vi "FTW-Example-SQLite.vi"() -> ()   [LabVIEW 2012]
uses:
  Core/src/Database/FTW-SQLite-DatabaseType.ctl
  Core/src/Time/FTW-Time-Uptime.vi
  Core/src/Database/FTW-SQLite-PrepareStatement.vi
  Core/src/Database/FTW-SQLite-LibraryFilepath.vi
  Core/src/Database/FTW-SQLite-LibraryReturnValue.vi
  Core/src/Error/FTW-ERR-ThrowImpossibleError.vi
  Core/utils/CodeGen/SQLite-Fetch/FTW-SQLite-Fetch.xnode
  Core/src/Database/FTW-SQLite-Connector.lvclass
  Core/src/Database/FTW-SQLite-AccessMode.ctl
panel:
  out "Result Set":cluster{"Year":string}[](array[cluster])
  out "Time to Compile SQL (Fetch)":dbl format="%.6fsec"
  out "Time to Execute+Compile (Fetch)":dbl format="%.6fsec"
  out "Time to Compile SQL (DDL)":dbl format="%.6fsec"
  out "Time to Execute+Compile (DDL)":dbl format="%.6fsec"
  out "Results from Database":T1(array[cluster])
  out "Data to put into Database":T2(array[cluster])
  out "error out":errorcluster
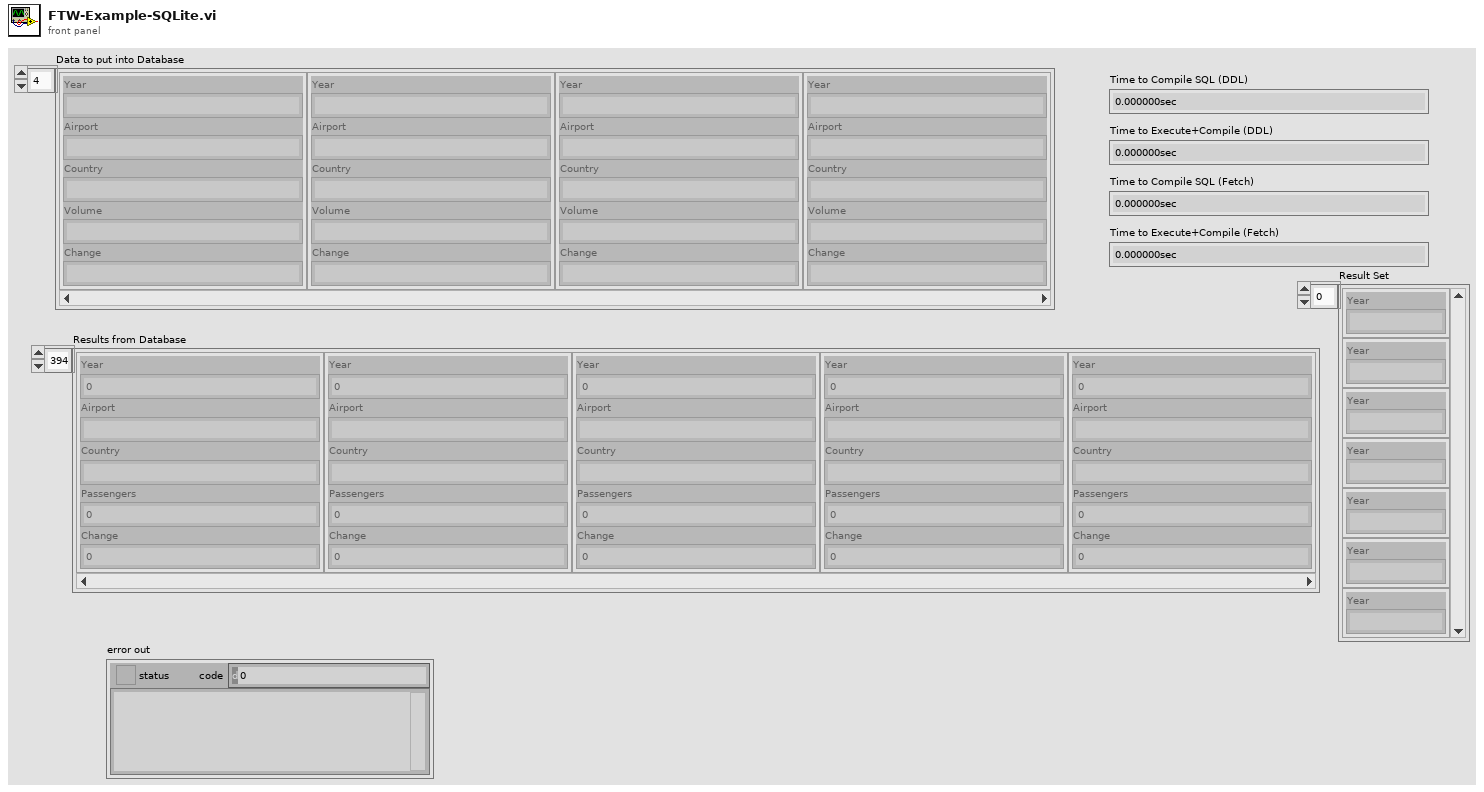
[diagram p1: front panel]
types:
  T1 = cluster{"Year":i32, "Airport":string, "Country":string, "Passengers":i32, "Change":dbl}[]
  T2 = cluster{"Year":string, "Airport":string, "Country":string, "Volume":string, "Change":string}[]
  T3 = cluster{"Year":i32, "Airport":string, "Country":string, "Passengers":i32, "Change":dbl}
  T4 = cluster{"Year":string, "Airport":string, "Country":string, "Volume":string, "Change":string}
  T5 = typedef "FTW-SQLite-Connector.lvclass/FTW-SQLite-DatabaseType.ctl" = enum16{"Disk", "Memory"}
  T6 = typedef "FTW-SQLite-Connector.lvclass/FTW-SQLite-AccessMode.ctl" = enum16{"Read", "Read/Write", "Read/Write/Create"}
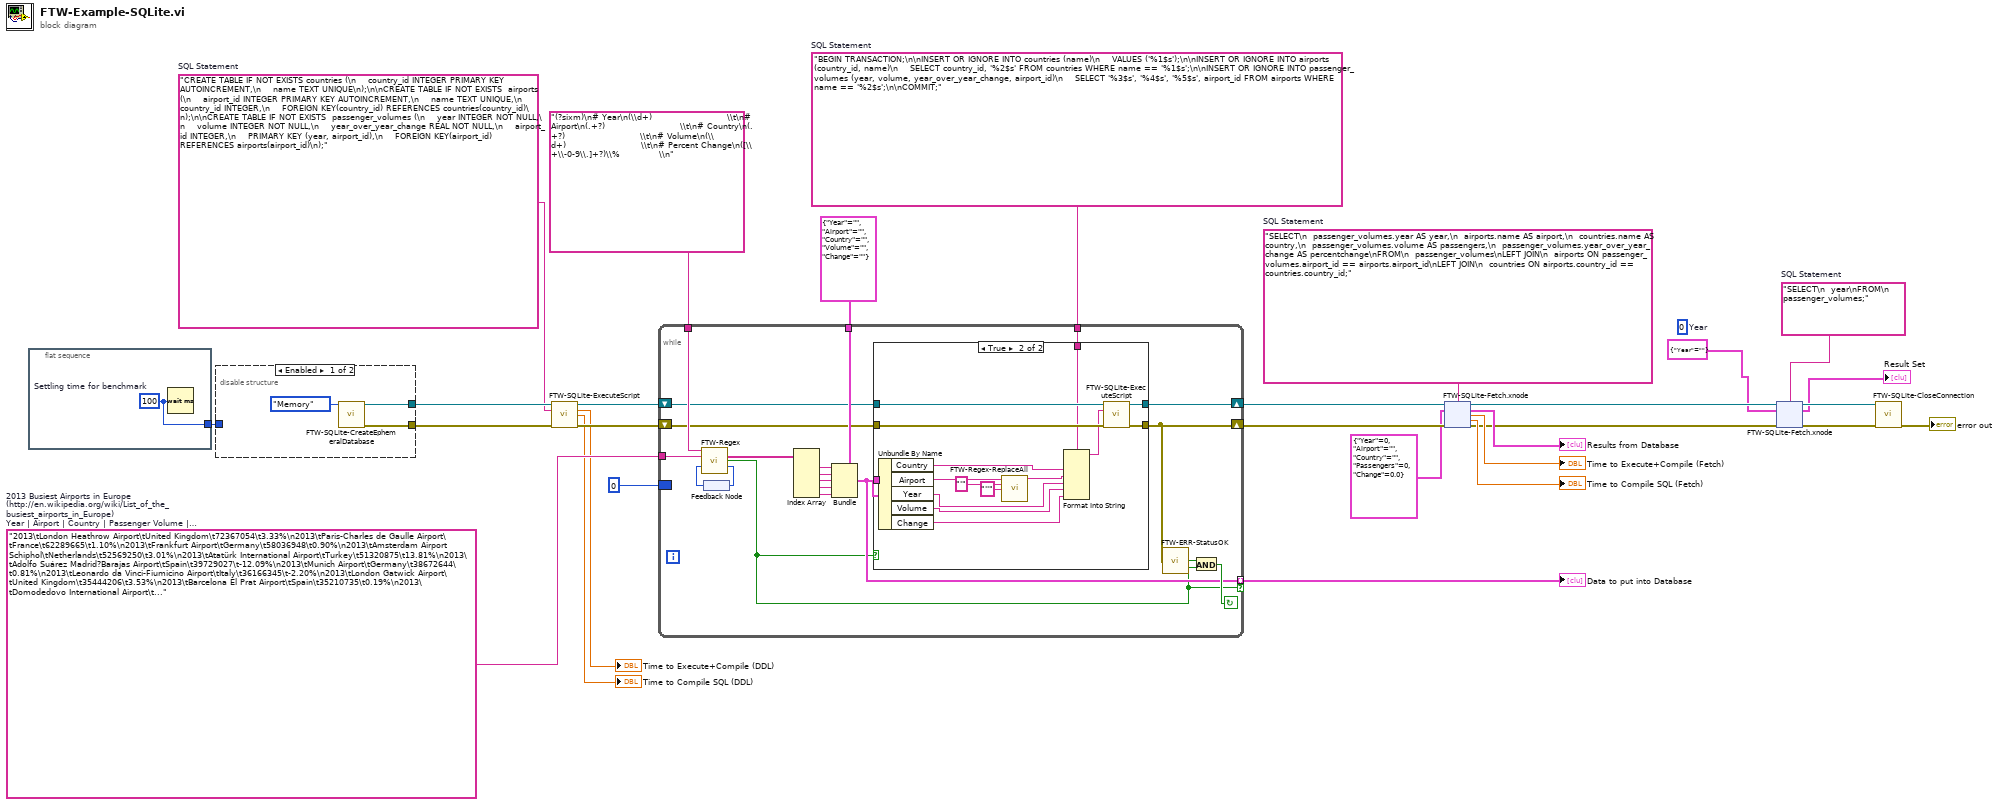
[diagram p0: block diagram]
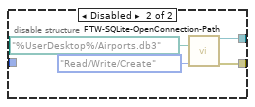
[diagram p2: hidden frame]
diagram:
  (unwired) 0  # Year
  w4 = "SELECT\n  year\nFROM\n  passenger_volumes;"  # SQL Statement
  w16 = "SELECT\n  passenger_volumes.year AS year,\n  airports.name AS airport,\n  countries.name AS country,\n  passenger_volumes.volume AS passengers,\n  passenger_volumes.year_over_year_change AS percentchange\nFROM\n  passenger_volumes\nLEFT JOIN\n  airports ON passenger_volumes.airport_id == airports.airport_id\nLEFT JOIN\n  countries ON airports.country_id == countries.country_id;"  # SQL Statement
  w19 = "BEGIN TRANSACTION;\n\nINSERT OR IGNORE INTO countries (name)\n    VALUES ('%1$s');\n\nINSERT OR IGNORE INTO airports (country_id, name)\n    SELECT country_id, '%2$s' FROM countries WHERE name == '%1$s';\n\nINSERT OR IGNORE INTO passenger_volumes (year, volume, year_over_year_change, airport_id)\n    SELECT '%3$s', '%4$s', '%5$s', airport_id FROM airports WHERE name == '%2$s';\n\nCOMMIT;"  # SQL Statement
  w25 = "2013\tLondon Heathrow Airport\tUnited Kingdom\t72367054\t3.33%\n2013\tParis-Charles de Gaulle Airport\tFrance\t62289665\t1.10%\n2013\tFrankfurt Airport\tGermany\t58036948\t0.90%\n2013\tAmsterdam Airport Schiphol\tNetherlands\t52569250\t3.01%\n2013\tAtatürk International Airport\tTurkey\t51320875\t13.81%\n2013\tAdolfo Suárez Madrid?Barajas Airport\tSpain\t39729027\t-12.09%\n2013\tMunich Airport\tGermany\t38672644\t0.81%\n2013\tLeonardo da Vinci-Fiumicino Airport\tItaly\t36166345\t-2.20%\n2013\tLondon Gatwick Airport\tUnited Kingdom\t35444206\t3.53%\n2013\tBarcelona El Prat Airport\tSpain\t35210735\t0.19%\n2013\tDomodedovo International Airport\tRussia\t30760000\t9.21%\n2013\tSheremetyevo International Airport\tRussia\t29256000\t12.38%\n2013\tParis-Orly Airport\tFrance\t28274154\t3.83%\n2013\tAntalya Airport\tTurkey\t27003712\t8.04%\n2013\tZürich Airport\tSwitzerland\t24865138\t0.25%\n2013\tCopenhagen Airport, Kastrup\tDenmark\t24067030\t3.13%\n2013\tOslo Gardermoen International Airport\tNorway\t22956540\t3.97%\n2013\tPalma de Mallorca Airport\tSpain\t22768082\t0.45%\n2013\tVienna International Airport\tAustria\t21999926\t-0.75%\n2013\tDüsseldorf International Airport\tGermany\t21228226\t1.90%\n2013\tManchester Airport\tUnited Kingdom\t20751581\t5.14%\n2013\tStockholm-Arlanda Airport\tSweden\t20681554\t5.29%\n2013\tDublin Airport\tIreland\t20200000\t5.76%\n2013\tBerlin Tegel Airport\tGermany\t19591838\t7.86%\n2013\tBrussels Airport\tBelgium\t19133222\t0.85%\n2013\tSabiha Gökçen Airport\tTurkey\t18641842\t28.68%\n2013\tMalpensa Airport\tItaly\t17955075\t-3.14%\n2013\tLondon Stansted Airport\tUnited Kingdom\t17852393\t2.17%\n2013\tLisbon Portela Airport\tPortugal\t16024955\t4.73%\n2013\tHelsinki-Vantaa Airport\tFinland\t15279043\t2.83%\n2013\tGeneva International Airport\tSwitzerland\t14436149\t3.86%\n2013\tHamburg Airport\tGermany\t13502553\t-1.42%\n2013\tMálaga Airport\tSpain\t12922403\t2.71%\n2013\tPulkovo Airport\tRussia\t12854366\t15.24%\n2013\tAthens International Airport\tGreece\t12460298\t-3.74%\n2013\tNice Côte d'Azur Airport\tFrance\t11554195\t3.26%\n2013\tVnukovo International Airport\tRussia\t11180000\t15.38%\n2013\tVáclav Havel Airport Prague\tCzech Republic\t10974196\t1.54%\n2013\tEsenbo?a International Airport\tTurkey\t10928403\t18.30%\n2013\tFrederic Chopin Airport\tPoland\t10683402\t11.43%\n2013\tAdnan Menderes Airport\tTurkey\t10208627\t9.11%\n2013\tEdinburgh Airport\tUnited Kingdom\t9775443\t6.31%\n2013\tGran Canaria Airport\tSpain\t9770253\t-1.23%\n2013\tLondon Luton Airport\tUnited Kingdom\t9697944\t0.83%\n2013\tAlicante Airport\tSpain\t9638860\t8.85%\n2013\tStuttgart Airport\tGermany\t9577551\t-1.47%\n2013\tBirmingham Airport\tUnited Kingdom\t9120201\t2.22%\n2013\tCologne Bonn Airport\tGermany\t9077346\t-2.18%\n2013\tLinate Airport\tItaly\t9034373\t-2.12%\n2013\tOrio al Serio Airport\tItaly\t8964376\t0.83%\n2013\tTenerife South Airport\tSpain\t8701983\t2.01%\n2013\tLyon-Saint Exupéry Airport\tFrance\t8562288\t1.32%\n2013\tBudapest Liszt Ferenc International Airport\tHungary\t8520880\t0.20%\n2013\tVenice Marco Polo Airport\tItaly\t8403790\t2.63%\n2013\tMarseille Provence Airport\tFrance\t8260619\t-0.42%\n2013\tBoryspil International Airport\tUkraine\t7930000\t-6.46%\n2013\tHenri Coand? International Airport\tRomania\t7649503\t7.44%\n2013\tBlagnac Airport\tFrance\t7567634\t0.11%\n2013\tGlasgow International Airport\tUnited Kingdom\t7363764\t2.88%\n2013\tBrussels South Charleroi Airport\tBelgium\t6786979\t4.15%\n2013\tBerlin Schönefeld Airport\tGermany\t6727306\t-5.21%\n2013\tCatania-Fontanarossa Airport\tItaly\t6400127\t2.45%\n2013\tFrancisco de Sá Carneiro Airport\tPortugal\t6370749\t5.30%\n2013\tBergen Flesland Airport\tNorway\t6213960\t6.87%\n2013\tBologna Airport\tItaly\t6193783\t3.95%\n2013\tBristol Airport\tUnited Kingdom\t6131896\t3.55%\n2013\tFaro Airport\tPortugal\t5978685\t5.40%\n2013\tEuroAirport Basel-Mulhouse-Freiburg\tSwitzerland-France-Germany\t5880771\t9.83%\n2013\tHeraklion International Airport\tGreece\t5792429\t15.52%\n2013\tIbiza Airport\tSpain\t5726581\t3.09%\n2013\tNaples Airport\tItaly\t5444422\t-6.16%\n2013\tLanzarote Airport\tSpain\t5334598\t3.21%\n2013\tLangenhagen Airport\tGermany\t5234909\t-1.00%\n2013\tGothenburg-Landvetter Airport\tSweden\t5004093\t3.07%\n2013\tLarnaca International Airport\tCyprus\t4863577\t-5.86%\n2013\tRiga International Airport\tLatvia\t4793213\t0.53%\n2013\tRome Ciampino Airport\tItaly\t4749251\t5.60%\n2013\tStavanger Sola Airport\tNorway\t4668403\t5.76%\n2013\tValencia Airport\tSpain\t4599990\t-3.20%\n2013\tBordeaux - Mérignac Airport\tFrance\t4574357\t4.43%\n2013\tGalileo Galilei Airport\tItaly\t4479690\t-0.34%\n2013\tNewcastle Airport\tUnited Kingdom\t4420839\t1.25%\n2013\tPalermo Airport\tItaly\t4349672\t-5.62%\n2013\tEast Midlands Airport\tUnited Kingdom\t4334117\t6.33%\n2013\tAdana ?akirpa?a Airport\tTurkey\t4316678\t14.28%\n2013\tTrondheim Værnes Airport\tNorway\t4311328\t3.63%\n2013\tKoltsovo Airport\tRussia\t4293002\t13.48%\n2013\tFuerteventura Airport\tSpain\t4259341\t-3.18%\n2013\tRhodes International Airport\tGreece\t4200068\t10.10%\n2013\tLiverpool John Lennon Airport\tUnited Kingdom\t4187493\t-6.18%\n2013\tThessaloniki International Airport, \"Macedonia\"\tGreece\t4085032\t1.05%\n2013\tDalaman Airport\tTurkey\t4057173\t6.49%\n2013\tMalta International Airport\tMalta\t4052000\t10.88%\n2013\tBelfast International Airport\tUnited Kingdom\t4023336\t-6.73%\n2013\tBeauvais-Tillé Airport\tFrance\t3952908\t2.34%\n2013\tNantes Atlantique Airport\tFrance\t3930849\t8.24%\n2013\tBilbao Airport\tSpain\t3800789\t-8.88%\n2013\tTolmachevo Airport\tRussia\t3748211\t14.74%\n2013\tSan Pablo Airport\tSpain\t3687727\t-14.08%\n2013\tKraków Airport\tPoland\t3647616\t6.07%\n2012\tLondon Heathrow Airport\tUnited Kingdom\t70037417\t0.87%\n2012\tParis-Charles de Gaulle Airport\tFrance\t61611934\t1.05%\n2012\tFrankfurt Airport\tGermany\t57520001\t1.92%\n2012\tAmsterdam Airport Schiphol\tNetherlands\t51035590\t2.57%\n2012\tMadrid?Barajas Airport\tSpain\t45190528\t-9.02%\n2012\tAtatürk International Airport\tTurkey\t45091962\t20.58%\n2012\tMunich Airport\tGermany\t38360604\t1.58%\n2012\tLeonardo da Vinci-Fiumicino Airport\tItaly\t36980911\t-1.78%\n2012\tBarcelona El Prat Airport\tSpain\t35144503\t2.17%\n2012\tLondon Gatwick Airport\tUnited Kingdom\t34235982\t1.67%\n2012\tDomodedovo International Airport\tRussia\t28165657\t9.59%\n2012\tParis-Orly Airport\tFrance\t27232263\t0.34%\n2012\tSheremetyevo International Airport\tRussia\t26032975\t16.47%\n2012\tAntalya Airport\tTurkey\t24993667\t-0.48%\n2012\tZürich Airport\tSwitzerland\t24802466\t1.91%\n2012\tCopenhagen Airport, Kastrup\tDenmark\t23336187\t2.69%\n2012\tPalma de Mallorca Airport\tSpain\t22666858\t-0.26%\n2012\tVienna International Airport\tAustria\t22165794\t5.02%\n2012\tOslo Gardermoen International Airport\tNorway\t22080433\t4.63%\n2012\tDüsseldorf International Airport\tGermany\t20833246\t2.43%\n2012\tManchester Airport\tUnited Kingdom\t19736502\t4.47%\n2012\tStockholm-Arlanda Airport\tSweden\t19642029\t3.00%\n2012\tDublin Airport\tIreland\t19099649\t1.91%\n2012\tBrussels Airport\tBelgium\t18971332\t0.99%\n2012\tMalpensa Airport\tItaly\t18537301\t-3.97%\n2012\tBerlin Tegel Airport\tGermany\t18164203\t7.35%\n2012\tLondon Stansted Airport\tUnited Kingdom\t17472699\t-3.21%\n2012\tLisbon Portela Airport\tPortugal\t15301176\t3.35%\n2012\tHelsinki Airport\tFinland\t14858215\t-0.05%\n2012\tSabiha Gökçen Airport\tTurkey\t14487242\t13.63%\n2012\tGeneva International Airport\tSwitzerland\t13899422\t6.01%\n2012\tHamburg Airport\tGermany\t13697402\t1.03%\n2012\tAthens International Airport\tGreece\t12944041\t-10.40%\n2012\tMálaga Airport\tSpain\t12581944\t-1.88%\n2012\tNice Côte d'Azur Airport\tFrance\t11189896\t7.37%\n2012\tPulkovo Airport\tRussia\t11154560\t16.06%\n2012\tVáclav Havel Airport Prague\tCzech Republic\t10807890\t-8.32%\n2012\tGran Canaria Airport\tSpain\t9892067\t-6.14%\n2012\tStuttgart Airport\tGermany\t9720877\t1.45%\n2012\tVnukovo International Airport\tRussia\t9690000\t18.21%\n2012\tLondon Luton Airport\tUnited Kingdom\t9617697\t1.09%\n2012\tFrederic Chopin Airport\tPoland\t9587842\t2.68%\n2012\tAdnan Menderes Airport\tTurkey\t9356284\t9.77%\n2012\tCologne Bonn Airport\tGermany\t9280070\t-3.57%\n2012\tEsenbo?a Airport\tTurkey\t9237886\t8.87%\n2012\tLinate Airport\tItaly\t9229890\t1.11%\n2012\tEdinburgh Airport\tUnited Kingdom\t9195061\t-2.03%\n2012\tBirmingham Airport\tUnited Kingdom\t8922539\t3.55%\n2012\tOrio al Serio Airport\tItaly\t8890720\t5.59%\n2012\tAlicante Airport\tSpain\t8855444\t-10.67%\n2012\tTenerife South Airport\tSpain\t8530729\t-1.45%\n2012\tBudapest Liszt Ferenc International Airport\tHungary\t8504020\t-4.67%\n2012\tBoryspil International Airport\tUkraine\t8478091\t5.36%\n2012\tLyon-Saint Exupéry Airport\tFrance\t8451039\t0.16%\n2012\tMarseille Provence Airport\tFrance\t8295479\t12.61%\n2012\tVenice Marco Polo Airport\tItaly\t8188455\t-4.62%\n2012\tBlagnac Airport\tFrance\t7559350\t8.17%\n2012\tGlasgow International Airport\tUnited Kingdom\t7157859\t4.04%\n2012\tHenri Coand? International Airport\tRomania\t7120067\t41.01%\n2012\tBerlin Schönefeld Airport\tGermany\t7097274\t-0.23%\n2012\tBrussels South Charleroi Airport\tBelgium\t6516427\t10.43%\n2012\tCatania-Fontanarossa Airport\tItaly\t6246888\t-8.05%\n2012\tFrancisco de Sá Carneiro Airport\tPortugal\t6050094\t0.76%\n2012\tBologna Airport\tItaly\t5958648\t1.24%\n2012\tBristol Airport\tUnited Kingdom\t5921530\t2.44%\n2012\tBergen Flesland Airport\tNorway\t5814413\t3.80%\n2012\tNaples Airport\tItaly\t5801836\t0.57%\n2012\tFaro Airport\tPortugal\t5672377\t1.01%\n2012\tIbiza Airport\tSpain\t5555048\t-1.56%\n2012\tEuroAirport Basel-Mulhouse-Freiburg\tSwitzerland-France-Germany\t5354674\t5.96%\n2012\tLangenhagen Airport\tGermany\t5287831\t-0.98%\n2012\tLanzarote Airport\tSpain\t5168775\t-6.76%\n2012\tLarnaca International Airport\tCyprus\t5166224\t-6.20%\n2012\tHeraklion International Airport\tGreece\t5014312\t-5.26%\n2012\tGothenburg-Landvetter Airport\tSweden\t4854888\t-1.05%\n2012\tRiga International Airport\tLatvia\t4767878\t-6.64%\n2012\tValencia Airport\tSpain\t4752020\t-4.57%\n2012\tPalermo Airport\tItaly\t4608533\t-7.70%\n2012\tRome Ciampino Airport\tItaly\t4497376\t-5.95%\n2012\tGalileo Galilei Airport\tItaly\t4494915\t-0.70%\n2012\tLiverpool John Lennon Airport\tUnited Kingdom\t4463257\t-15.00%\n2012\tStavanger Sola Airport\tNorway\t4413987\t6.83%\n2012\tFuerteventura Airport\tSpain\t4399023\t-11.10%\n2012\tBordeaux - Mérignac Airport\tFrance\t4380145\t6.38%\n2012\tNewcastle Airport\tUnited Kingdom\t4366196\t0.46%\n2012\tBelfast International Airport\tUnited Kingdom\t4313685\t5.12%\n2012\tSan Pablo Airport\tSpain\t4292020\t-13.46%\n2012\tBilbao Airport\tSpain\t4171065\t3.09%\n2012\tTrondheim Værnes Airport\tNorway\t4160162\t5.95%\n2012\tEast Midlands Airport\tUnited Kingdom\t4076178\t-3.30%\n2012\tThessaloniki International Airport, \"Macedonia\"\tGreece\t4042539\t-0.47%\n2012\tBeauvais-Tillé Airport\tFrance\t3862431\t5.02%\n2012\tRhodes International Airport\tGreece\t3814706\t-8.06%\n2012\tDalaman Airport\tTurkey\t3810015\t2.06%\n2012\tKoltsovo Airport\tRussia\t3783069\t12.73%\n2012\tBari Airport\tItaly\t3780112\t1.46%\n2012\tAdana ?akirpa?a Airport\tTurkey\t3777348\t16.55%\n2012\tLos Rodeos Airport\tSpain\t3717944\t-9.21%\n2012\tMalta International Airport\tMalta\t3654283\t4.10%\n2012\tNantes Atlantique Airport\tFrance\t3631693\t11.88%\n2011\tLondon Heathrow Airport\tUnited Kingdom\t69433230\t5.39%\n2011\tParis-Charles de Gaulle Airport\tFrance\t60970551\t4.82%\n2011\tFrankfurt Airport\tGermany\t56436255\t6.46%\n2011\tAmsterdam Airport Schiphol\tNetherlands\t49755252\t10.05%\n2011\tMadrid Barajas Airport\tSpain\t49671270\t-0.39%\n2011\tMunich Airport\tGermany\t37763701\t8.76%\n2011\tRome-Fiumicino Airport\tItaly\t37651700\t3.62%\n2011\tAtatürk International Airport\tTurkey\t37394694\t16.34%\n2011\tBarcelona El Prat Airport\tSpain\t34398226\t17.76%\n2011\tLondon Gatwick Airport\tUnited Kingdom\t33674264\t7.33%\n2011\tParis-Orly Airport\tFrance\t27139076\t7.68%\n2011\tDomodedovo International Airport\tRussia\t25701610\t15.49%\n2011\tAntalya Airport\tTurkey\t25113635\t14.09%\n2011\tZurich Airport\tSwitzerland\t24337954\t6.38%\n2011\tPalma de Mallorca Airport\tSpain\t22726707\t7.62%\n2011\tCopenhagen Airport\tDenmark\t22725517\t5.69%\n2011\tSheremetyevo International Airport\tRussia\t22351317\t16.88%\n2011\tVienna International Airport\tAustria\t21106292\t7.19%\n2011\tOslo-Gardermoen Airport\tNorway\t21103623\t10.54%\n2011\tDüsseldorf International Airport\tGermany\t20339466\t7.12%\n2011\tMilan Malpensa Airport\tItaly\t19303131\t1.88%\n2011\tStockholm-Arlanda Airport\tSweden\t19069065\t12.42%\n2011\tManchester Airport\tUnited Kingdom\t18892756\t6.38%\n2011\tBrussels Airport\tBelgium\t18786034\t9.34%\n2011\tDublin Airport\tIreland\t18740593\t1.68%\n2011\tLondon Stansted Airport\tUnited Kingdom\t18052843\t-2.80%\n2011\tBerlin Tegel Airport\tGermany\t16919820\t12.61%\n2011\tHelsinki Airport\tFinland\t14865871\t15.39%\n2011\tLisbon Portela Airport\tPortugal\t14805624\t5.49%\n2011\tAthens International Airport\tGreece\t14446963\t-5.59%\n2011\tHamburg Airport\tGermany\t13558261\t4.60%\n2011\tGeneva Cointrin International Airport\tSwitzerland\t13111741\t11.25%\n2011\tMálaga Airport\tSpain\t12823117\t6.29%\n2011\tSabiha Gökçen Airport\tTurkey\t12749230\t13.94%\n2011\tVáclav Havel Airport Prague\tCzech Republic\t11788629\t2.01%\n2011\tGran Canaria Airport\tSpain\t10538829\t11.10%\n2011\tNice Côte d'Azur Airport\tFrance\t10422073\t8.53%\n2011\tAlicante Airport\tSpain\t9913731\t5.66%\n2011\tCologne Bonn Airport\tGermany\t9623398\t-2.30%\n2011\tPulkovo Airport\tRussia\t9610767\t14.53%\n2011\tStuttgart Airport\tGermany\t9582265\t3.95%\n2011\tLondon Luton Airport\tUnited Kingdom\t9513704\t8.87%\n2011\tEdinburgh Airport\tUnited Kingdom\t9385245\t9.17%\n2011\tFrederic Chopin Airport\tPoland\t9337734\t7.18%\n2011\tMilan Linate Airport\tItaly\t9128522\t10.03%\n2011\tBudapest Liszt Ferenc International Airport\tHungary\t8920653\t8.92%\n2011\tTenerife South Airport\tSpain\t8656487\t17.63%\n2011\tBirmingham Airport\tUnited Kingdom\t8616296\t0.51%\n2011\tVenice Marco Polo Airport\tItaly\t8584651\t25.24%\n2011\tAdnan Menderes Airport\tTurkey\t8523533\t13.87%\n2011\tEsenbo?a Airport\tTurkey\t8485467\t9.29%\n2011\tLyon-Saint Exupéry Airport\tFrance\t8437141\t5.74%\n2011\tBergamo Orio al Serio airport\tItaly\t8419948\t9.67%\n2011\tVnukovo International Airport\tRussia\t8197162\t-13.35%\n2011\tBoryspil International Airport\tUkraine\t8047115\t20.24%\n2011\tMarseille Provence Airport\tFrance\t7366873\t-2.10%\n2011\tBerlin Schönefeld Airport\tGermany\t7113989\t-2.52%\n2011\tBlagnac Airport\tFrance\t6988140\t9.09%\n2011\tGlasgow International Airport\tUnited Kingdom\t6880217\t5.06%\n2011\tCatania-Fontanarossa Airport\tItaly\t6794063\t7.53%\n2011\tFrancisco de Sá Carneiro Airport\tPortugal\t6004589\t13.74%\n2011\tBrussels South Charleroi Airport\tBelgium\t5901007\t13.58%\n2011\tBologna Airport\tItaly\t5885884\t6.96%\n2011\tBristol Airport\tUnited Kingdom\t5780746\t0.58%\n2011\tNaples Airport\tItaly\t5768873\t3.54%\n2011\tIbiza Airport\tSpain\t5643180\t11.95%\n2011\tFaro Airport\tPortugal\t5615580\t5.24%\n2011\tBergen Airport\tNorway\t5814413\t14.50%\n2011\tLanzarote Airport\tSpain\t5543744\t12.26%\n2011\tLarnaca International Airport\tCyprus\t5507762\t2.61%\n2011\tLangenhagen Airport\tGermany\t5340264\t5.54%\n2011\tHeraklion International Airport\tGreece\t5292687\t7.85%\n2011\tLiverpool John Lennon Airport\tUnited Kingdom\t5251161\t4.73%\n2011\tRiga International Airport\tLatvia\t5106926\t9.50%\n2011\tEuroAirport Basel-Mulhouse-Freiburg\tSwitzerland-France-Germany\t5053664\t22.39%\n2011\tHenri Coand? International Airport\tRomania\t5049443\t2.67%\n2011\tPalermo Airport\tItaly\t4992798\t14.96%\n2011\tValencia Airport\tSpain\t4979511\t0.92%\n2011\tSan Pablo Airport\tSpain\t4959359\t17.39%\n2011\tFuerteventura Airport\tSpain\t4948018\t18.56%\n2011\tGothenburg-Landvetter Airport\tSweden\t4906639\t18.71%\n2011\tRome Ciampino Airport\tItaly\t4781731\t5.51%\n2011\tPisa Airport\tItaly\t4526723\t11.52%\n2011\tNewcastle Airport\tUnited Kingdom\t4346270\t-0.23%\n2011\tEast Midlands Airport\tUnited Kingdom\t4215192\t2.47%\n2011\tRhodes International Airport\tGreece\t4149274\t15.69%\n2011\tStavanger Airport\tNorway\t4131974\t12.44%\n2011\tBordeaux - Mérignac Airport\tFrance\t4117303\t12.38%\n2011\tBelfast International Airport\tUnited Kingdom\t4103620\t2.18%\n2011\tLos Rodeos Airport\tSpain\t4095103\t1.08%\n2011\tThessaloniki International Airport, \"Macedonia\"\tGreece\t4061697\t3.86%\n2011\tBilbao Airport\tSpain\t4046172\t4.04%\n2011\tNuremberg Airport\tGermany\t3962617\t-2.61%\n2011\tTrondheim Airport\tNorway\t3926461\t11.49%\n2011\tDalaman Airport\tTurkey\t3732941\t-1.40%\n2011\tBari Airport\tItaly\t3725629\t9.64%\n2011\tTurin Airport\tItaly\t3710485\t4.45%\n2011\tCagliari-Elmas Airport\tItaly\t3698982\t7.43%\n2011\tBeauvais-Tillé Airport\tFrance\t3677825\t25.45%\n2011\tMalta International Airport\tMalta\t3510213\t6.36%\n2010\tLondon Heathrow Airport\tUnited Kingdom\t65881660\t-0.24%\n2010\tParis-Charles de Gaulle Airport\tFrance\t58164612\t0.45%\n2010\tFrankfurt Airport\tGermany\t53009221\t4.08%\n2010\tBarajas Airport\tSpain\t49866113\t2.95%\n2010\tAmsterdam Airport Schiphol\tNetherlands\t45211749\t3.77%\n2010\tLeonardo da Vinci-Fiumicino Airport\tItaly\t36337050\t7.48%\n2010\tMunich Airport\tGermany\t34721605\t6.24%\n2010\tAtatürk International Airport\tTurkey\t32143819\t7.82%\n2010\tGatwick Airport\tUnited Kingdom\t31375290\t-3.14%\n2010\tBarcelona El Prat Airport\tSpain\t29209536\t6.52%\n2010\tParis-Orly Airport\tFrance\t25203969\t0.38%\n2010\tZurich Airport\tSwitzerland\t22878251\t4.34%\n2010\tDomodedovo International Airport\tRussia\t22253529\t19.16%\n2010\tAntalya Airport\tTurkey\t22013027\t19.99%\n2010\tCopenhagen Airport\tDenmark\t21501750\t9.06%\n2010\tPalma de Mallorca Airport\tSpain\t21117417\t-0.40%\n2010\tVienna International Airport\tAustria\t19691206\t8.71%\n2010\tSheremetyevo International Airport\tRussia\t19123007\t29.52%\n2010\tOslo-Gardermoen Airport\tNorway\t19091036\t5.55%\n2010\tDüsseldorf International Airport\tGermany\t18988149\t6.71%\n2010\tMalpensa Airport\tItaly\t18947808\t7.95%\n2010\tLondon Stansted Airport\tUnited Kingdom\t18573592\t-6.93%\n2010\tDublin Airport\tIreland\t18431064\t-10.11%\n2010\tManchester Airport\tUnited Kingdom\t17759173\t-5.16%\n2010\tBrussels Airport\tBelgium\t17180606\t1.07%\n2010\tStockholm-Arlanda Airport\tSweden\t16962416\t5.59%\n2010\tAthens International Airport\tGreece\t15303127\t-5.69%\n2010\tBerlin Tegel Airport\tGermany\t15025600\t5.96%\n2010\tLisbon Portela Airport\tPortugal\t14035273\t5.70%\n2010\tHamburg Airport\tGermany\t12962429\t5.99%\n2010\tHelsinki Airport\tFinland\t12883399\t2.32%\n2010\tMálaga Airport\tSpain\t12064521\t3.80%\n2010\tGeneva Cointrin International Airport\tSwitzerland\t11785522\t4.07%\n2010\tRuzyn? Airport\tCzech Republic\t11556858\t-0.74%\n2010\tSabiha Gökçen Airport\tTurkey\t11189678\t68.51%\n2010\tCologne Bonn Airport\tGermany\t9849779\t1.13%\n2010\tNice Côte d'Azur Airport\tFrance\t9603014\t-2.32%\n2010\tGran Canaria Airport\tSpain\t9486035\t3.61%\n2010\tVnukovo International Airport\tRussia\t9460292\t22.37%\n2010\tAlicante Airport\tSpain\t9382931\t2.66%\n2010\tStuttgart Airport\tGermany\t9218095\t3.17%\n2010\tLondon Luton Airport\tUnited Kingdom\t8738712\t-4.19%\n2010\tFrederic Chopin Airport\tPoland\t8712384\t4.70%\n2010\tEdinburgh Airport\tUnited Kingdom\t8596715\t-5.00%\n2010\tBirmingham Airport\tUnited Kingdom\t8572398\t-5.83%\n2010\tPulkovo Airport\tRussia\t8391281\t24.17%\n2010\tLinate Airport\tItaly\t8296450\t0.02%\n2010\tBudapest Liszt Ferenc International Airport\tHungary\t8190089\t1.17%\n2010\tLyon-Saint Exupéry Airport\tFrance\t7979228\t3.39%\n2010\tEsenbo?a Airport\tTurkey\t7763914\t27.60%\n2010\tOrio al Serio Airport\tItaly\t7677224\t7.26%\n2010\tMarseille Provence Airport\tFrance\t7524886\t3.22%\n2010\tAdnan Menderes Airport\tTurkey\t7485098\t20.69%\n2010\tTenerife South Airport\tSpain\t7358986\t3.53%\n2010\tBerlin Schönefeld Airport\tGermany\t7297911\t7.37%\n2010\tVenice Marco Polo Airport\tItaly\t6854595\t2.28%\n2010\tBoryspil International Airport\tUkraine\t6692382\t15.49%\n2010\tGlasgow International Airport\tUnited Kingdom\t6548865\t-9.36%\n2010\tBlagnac Airport\tFrance\t6405906\t2.04%\n2010\tCatania-Fontanarossa Airport\tItaly\t6318177\t6.52%\n2010\tBristol Airport\tUnited Kingdom\t5747604\t1.86%\n2010\tNaples Airport\tItaly\t5571738\t4.91%\n2010\tBologna Airport\tItaly\t5503106\t15.26%\n2010\tLarnaca International Airport\tCyprus\t5367724\t3.85%\n2010\tFaro Airport\tPortugal\t5336173\t5.31%\n2010\tFrancisco de Sá Carneiro Airport\tPortugal\t5279362\t17.08%\n2010\tBrussels South Charleroi Airport\tBelgium\t5195372\t31.96%\n2010\tBergen Airport\tNorway\t5078267\t4.43%\n2010\tLangenhagen Airport\tGermany\t5059800\t1.81%\n2010\tIbiza Airport\tSpain\t5040800\t10.23%\n2010\tLiverpool John Lennon Airport\tUnited Kingdom\t5013940\t2.65%\n2010\tLanzarote Airport\tSpain\t4938343\t5.03%\n2010\tValencia Airport\tSpain\t4934268\t3.90%\n2010\tHenri Coand? International Airport\tRomania\t4917952\t9.69%\n2010\tHeraklion International Airport\tGreece\t4907337\t-2.88%\n2010\tGirona-Costa Brava Airport\tSpain\t4863954\t-8.00%\n2010\tRiga International Airport\tLatvia\t4663647\t14.67%\n2010\tRome Ciampino Airport\tItaly\t4531834\t-4.75%\n2010\tNewcastle Airport\tUnited Kingdom\t4356130\t-5.05%\n2010\tPalermo Airport\tItaly\t4343227\t-0.17%\n2010\tSan Pablo Airport\tSpain\t4224718\t4.28%\n2010\tFuerteventura Airport\tSpain\t4173590\t11.64%\n2010\tGothenburg-Landvetter Airport\tSweden\t4133299\t12.04%\n2010\tEuroAirport Basel-Mulhouse-Freiburg\tSwitzerland-France-Germany\t4129186\t7.24%\n2010\tEast Midlands Airport\tUnited Kingdom\t4113501\t-11.69%\n2010\tNuremberg Airport\tGermany\t4068799\t2.60%\n2010\tGalileo Galilei Airport\tItaly\t4058957\t1.18%\n2010\tLos Rodeos Airport\tSpain\t4051356\t-0.07%\n2010\tBelfast International Airport\tUnited Kingdom\t4016170\t-11.66%\n2010\tThessaloniki International Airport, \"Macedonia\"\tGreece\t3910751\t-4.71%\n2010\tBilbao Airport\tSpain\t3888955\t6.40%\n2010\tDalaman Airport\tTurkey\t3785779\t5.22%\n2010\tStavanger Airport\tNorway\t3674816\t1.57%\n2010\tBordeaux - Mérignac Airport\tFrance\t3663702\t10.42%\n2010\tRhodes International Airport\tGreece\t3586572\t3.36%\n2010\tTurin Airport\tItaly\t3552519\t10.31%\n2010\tTrondheim Airport\tNorway\t3521734\t2.83%\n2010\tFrankfurt-Hahn Airport\tGermany\t3493451\t-7.91%\n2010\tCagliari-Elmas Airport\tItaly\t3438298\t3.28%\n2010\tBari Airport\tItaly\t3398110\t20.27%\n"  # 2013 Busiest Airports in Europe (http://en.wikipedia.org/wiki/List_of_the_busiest_airports_in_Europe) Year | Airport | Country | Passenger Volume | Percent Change over Previous Year
  w26 = "CREATE TABLE IF NOT EXISTS countries (\n    country_id INTEGER PRIMARY KEY AUTOINCREMENT,\n    name TEXT UNIQUE\n);\n\nCREATE TABLE IF NOT EXISTS  airports (\n    airport_id INTEGER PRIMARY KEY AUTOINCREMENT,\n    name TEXT UNIQUE,\n    country_id INTEGER,\n    FOREIGN KEY(country_id) REFERENCES countries(country_id)\n);\n\nCREATE TABLE IF NOT EXISTS  passenger_volumes (\n    year INTEGER NOT NULL,\n    volume INTEGER NOT NULL,\n    year_over_year_change REAL NOT NULL,\n    airport_id INTEGER,\n    PRIMARY KEY (year, airport_id),\n    FOREIGN KEY(airport_id) REFERENCES airports(airport_id)\n);"  # SQL Statement
  n1 = flat-sequence {
    tunnel: [w30] -> w9
    frame #0 {
      w30 = u32 100  # Settling time for benchmark
      n2 = Wait (ms)(milliseconds to wait=w30) -> ()  [unwired: 1 out]
    }
  }
  n3 = disable-structure shown="Enabled" {
    disable-tunnel: [w32 w36] -> w28
    disable-tunnel: [w31 w37] -> w27
    disable-tunnel: w9 -> [_ _]
    frame Enabled {
      n4 = call "FTW-SQLite-CreateEphemeralDatabase.vi"("Database Type"=FTW-SQLite-DatabaseType."Memory") -> ("SQLite Connector"=w31:refnum<class "FTW-SQLite-Connector.lvclass">, "error out"=w32:errorcluster)  [unwired: 13 in]
    }
    frame Disabled {
      n5 = call "FTW-SQLite-OpenConnection-Path.vi"("Database Filepath"=path "%UserDesktop%/Airports.db3", "Access Mode"=FTW-SQLite-AccessMode."Read/Write/Create") -> ("SQLite Connector"=w37:refnum<class "FTW-SQLite-Connector.lvclass">, "error out"=w36:errorcluster)  [unwired: 12 in]
    }
  }
  n6 = call "FTW-SQLite-ExecuteScript.vi"("SQLite Connector"=w27, "SQL Script"=w26, "error in"=w28) -> ("SQLite Connector out"=w21:refnum<class "FTW-SQLite-Connector.lvclass">, "Time to Execute+Compile"=→"Time to Execute+Compile (DDL)":dbl, "Time to Compile SQL"=→"Time to Compile SQL (DDL)":dbl, "error out"=w20:errorcluster)  [unwired: 9 in]
  n7 = while {
    tunnel: w25 -> [w57]
    tunnel: T4 {"Year"="", "Airport"="", "Country"="", "Volume"="", "Change"=""} -> [w53]
    tunnel: "(?sixm)\n# Year\n(\\d+)                         \\t\n# Airport\n(.+?)                         \\t\n# Country\n(.+?)                         \\t\n# Volume\n(\\d+)                         \\t\n# Percent Change\n([\\+\\-0-9\\.]+?)\\%             \\n" ("Regular Expression") -> [w47]
    border: 0 ("Offset after Match") -> [_]
    shift-right: [w45] -> w17
    shift-left: w21 -> [w46]
    shift-right: [w42] -> w15
    shift-left: w20 -> [w44]
    tunnel: w19 -> [w43]
    tunnel: [w39] -> w18 mode=indexing if=w38
    stop <- w40 continue-if-true
    n8 = feedback #1() -> (w56:i32)
    n9 = call "FTW-Regex.vi"("Regular Expression"=w47, "Input String"=w57, "Starting Offset"=w56) -> ("Submatches"=w54:string[], "Match Found?"=w38:bool, "Offset after Match"=w55:i32)  [unwired: 8 in, 2 out]
    n10 = feedback-in #1(w55) -> ()
    n11 = Index Array(array=w54) -> (element #1=w52:string, element #2=w51:string, element #3=w50:string, element #4=w49:string, element #5=w48:string)  [unwired: 5 in]
    n12 = Bundle(cluster=w53, "Year"=w52, "Airport"=w51, "Country"=w50, "Volume"=w49, "Change"=w48) -> (w39:T4)
    n13 = case shown="True" w38 {
      tunnel: w46 -> [w59 w74]
      tunnel: [w59 w73] -> w45
      tunnel: [w58 w72] -> w42
      tunnel: w44 -> [w58 w71]
      tunnel: w39 -> [_ w70]
      tunnel: w43 -> [_ w67]
      frame False {
      }
      frame True {
        n14 = Unbundle By Name(w70) -> ("Country"=w69:string, "Airport"=w66:string, "Year"=w62:string, "Volume"=w61:string, "Change"=w60:string)
        n15 = call "FTW-Regex-ReplaceAll.vi"("String"=w66, "Search for (Regular Expression)"="'", "Replace with"="''") -> ("String out"=w65:string)  [unwired: 10 in, 2 out]
        n16 = Format Into String(format string=w67, w69, w65, w62, w61, w60) -> (resulting string=w68:string)  [unwired: 2 in, 1 out]
        n17 = call "FTW-SQLite-ExecuteScript.vi"("SQLite Connector"=w74, "SQL Script"=w68, "error in"=w71) -> ("SQLite Connector out"=w73:refnum<class "FTW-SQLite-Connector.lvclass">, "error out"=w72:errorcluster)  [unwired: 9 in, 2 out]
      }
    }
    n18 = call "FTW-ERR-StatusOK.vi"("error to check"=w42) -> ("Status OK?"=w41:bool)
    n19 = And(x=w41, y=w38) -> (x .and. y?=w40:bool)
  }
  "Data to put into Database" <- w18
  n20 = xnode "FTW-SQLite-Fetch.xnode"("SQLite Connector"=w17, "SQL Script"=w16, "Row Datatype"=T3 {"Year"=0, "Airport"="", "Country"="", "Passengers"=0, "Change"=0.0}, "error in"=w15) -> ("SQLite Connector out"=w8:refnum<class "FTW-SQLite-Connector.lvclass">, "Result Set"=→"Results from Database":T1, "Time to Execute+Compile"=→"Time to Execute+Compile (Fetch)":dbl, "Time to Compile SQL"=→"Time to Compile SQL (Fetch)":dbl, "error out"=w6:errorcluster)
  n21 = xnode "FTW-SQLite-Fetch.xnode"("SQLite Connector"=w8, "SQL Script"=w4, "Row Datatype"=cluster{"Year":string} {"Year"=""}, "error in"=w6) -> ("SQLite Connector out"=w7:refnum<class "FTW-SQLite-Connector.lvclass">, "Result Set"=→"Result Set":cluster{"Year":string}[], "error out"=w5:errorcluster)  [unwired: 2 out]
  n22 = call "FTW-SQLite-CloseConnection.vi"("SQLite Connector"=w7, "error in"=w5) -> ("error out"=→"error out":errorcluster)  [unwired: 13 in]
